vi "subXMLGetPackageSourceIDs.vi"(11 "Refnum in":refnum<k20>) -> (3 "IDs":string[](array[string]))   [LabVIEW 2019, in "SolutionBuilder.lvlib" / "SolutionBuilder.lvclass"]
uses:
  SolutionBuilder.lvclass
  <vilib>/xml/NI_XML.lvlib
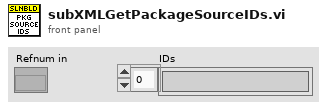
[diagram p1: front panel]
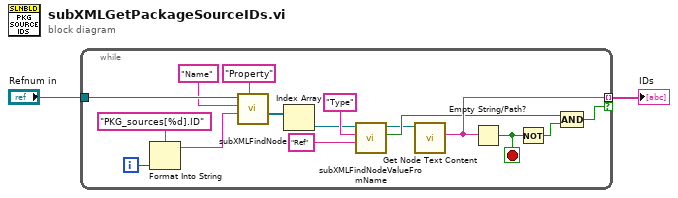
[diagram p0: block diagram]
diagram:
  n1 = while {
    tunnel: [w18] -> w2 mode=indexing if=w14
    tunnel: "Refnum in" -> [w16]
    i -> [w12]
    stop <- w17 stop-if-true
    n2 = Format Into String(format string="PKG_sources[%d].ID" ("Property value"), w12) -> (resulting string=w7:string)  [unwired: 2 in, 1 out]
    n3 = call "subXMLFindNode.vi"("Node name"="Property", "Property value"=w7, "Property name"="Name", "Refnum in"=w16) -> ("Nodes"=w3:refnum<k20>[])  [unwired: 6 in, 1 out]
    n4 = Index Array(array=w3) -> (element=w9:refnum<k20>)  [unwired: 1 in]
    n5 = call "subXMLFindNodeValueFromName.vi"("Property value"="Ref" ("Property name"), "Property name"="Type", "Refnum in"=w9) -> ("Found?"=w13:bool, "Refnum out"=w8:refnum<k20>)  [unwired: 6 in, 1 out]
    n6 = call <vilib>:"Get Node Text Content.vi"("node in"=w8) -> ("node text"=w18:string)  [unwired: 8 in, 2 out]
    n7 = Empty String/Path?(string/path=w18) -> (empty?=w17:bool)
    n8 = Not(x=w17) -> (.not. x?=w15:bool)
    n9 = Compound Arithmetic op=AND(w13, w15) -> (w14:bool)
  }
  "IDs" <- w2
